vi "Autonomous Independent.vi"() -> ()   [LabVIEW 2012]
doc: "This VI is called when autonomous begins, and will automatically be terminated when autonomous ends. You can carry out timed or sensor driven robot movement independently without needing to return to the caller."
uses:
  <vilib>/Rock Robotics/WPI/Relay/WPI_RelayValue.ctl
  <vilib>/Rock Robotics/WPI/Solenoid/WPI_SolenoidValue.ctl
  Robot Global Data.vi
  <vilib>/Rock Robotics/WPI/RobotDrive/WPI_RobotDriveGetSetRefNum.vi
  <vilib>/Rock Robotics/WPI/Solenoid/WPI_SolenoidSetEnum.vi
  <vilib>/Rock Robotics/WPI/Joystick/WPI_JoystickGetSetRefNum.vi
panel:
  in  "Auton Launch Reduction":dbl
  in  "Quicklaunch State":T1(ring)
  in  "Fast-Slow Variable":dbl=1.0
  out "Launch Wait tick":dbl
  out "Time Between tick":dbl
  out "Charge Up tick":dbl
  in  "Time Between Launches":dbl=2000.0
  in  "Charge Up Time":dbl=4000.0
  in  "Launch Wait Time":dbl=500.0
  in  "Drive wait time corner":dbl
  in  "Drive wait time middle":dbl
  out "Field Position":enum16{"Corner", "Middle"}(ring)
  in  "Numeric 0":dbl
  out "Current Movement, for debugging":T2 {"Y Joystick Value" scale=1.0..-1.0; "X Joystick Value" scale=-1.0..1.0}
  in  "Array of robot movements":T3(array[cluster]) {"Y Joystick Value" scale=1.0..-1.0; "X Joystick Value" scale=-1.0..1.0}
  # "Be sure to right-click and choose Data Operations>>Make Current Value default if you want to save the array values with the VI"
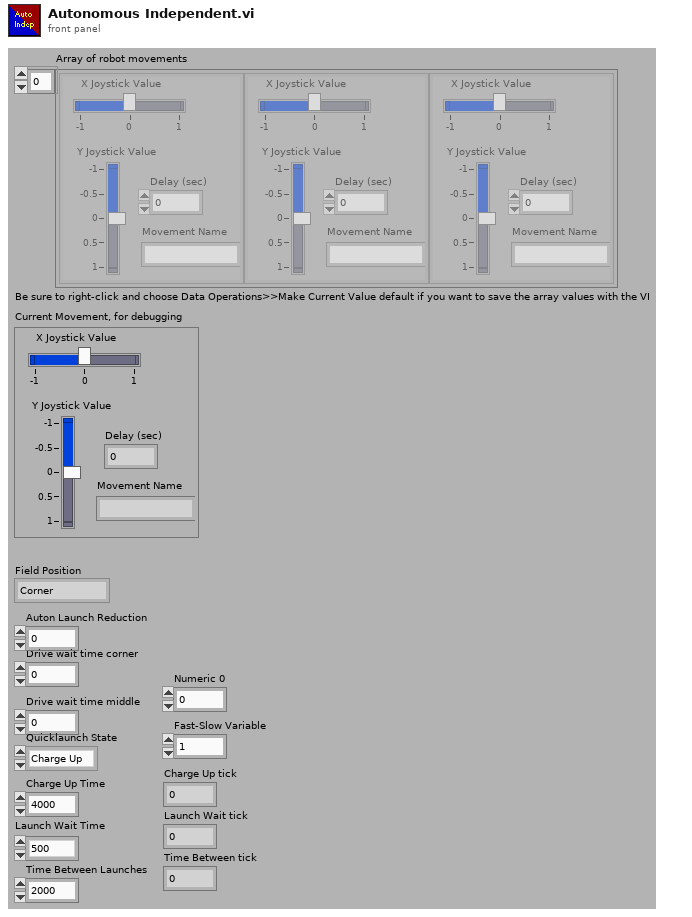
[diagram p1: front panel]
types:
  T1 = enum16{"Charge Up ", "Fire 1", "wait1", "Fire 2", "wait2", "Fire 3", "wait3", "Fire 4"}
  T2 = cluster{"X Joystick Value":dbl, "Y Joystick Value":dbl, "Delay (sec)":dbl, "Movement Name":string}
  T3 = cluster{"X Joystick Value":dbl, "Y Joystick Value":dbl, "Delay (sec)":dbl, "Movement Name":string}[]
  T4 = typedef "WPI_JoystickDevRef.ctl" = cluster{"Device":T5}
  T5 = typedef "WPI_JoystickDeviceEnum.ctl" = enum16{"USB 1", "USB 2", "USB 3", "USB 4", "Kinect 1", "Kinect 2"}
  T6 = cluster{"axis 1 (x)":dbl, "axis 2 (y)":dbl, "axis 3 (throttle)":dbl, "axis 4":dbl, "axis 5":dbl, "axis 6":dbl}
  T7 = typedef "WPI_SolenoidValue.ctl" = enum16{"Off", "On", "Forward", "Reverse"}
  T8 = typedef "WPI_RobotDriveDevRef.ctl" = cluster{"DevStatus":errorcluster, "Motors[]":T9[], "Square Inputs":bool, "Max Output":dbl, "Isochronous":bool}
  T9 = typedef "WPI_MotorControlDeviceRef.ctl" = cluster{"DeviceStatus":errorcluster, "Type":enum16{"PWM", "CAN"}, "PWM":cluster{"Digital Module":T10, "PWM Channel":T11, "DeadBand":T12}, "CAN":cluster{"Device Number":u8, "Control Mode":T13, "Semaphore":T14, "Max Vout":dbl}, "Invert":bool, "TransformRef":T15, "InvTransformRef":T15}
  T10 = typedef "FPGA_TypedefDigitalModule.ctl" = enum16{"Digital Module 1", "Digital Module 2"}
  T11 = typedef "FPGA_DIOPWMChannel.ctl" = enum8{"PWM 1", "PWM 2", "PWM 3", "PWM 4", "PWM 5", "PWM 6", "PWM 7", "PWM 8", "PWM 9", "PWM 10", "Invalid"}
  T12 = typedef "WPI_PWMDeadband.ctl" = cluster{"Name":string, "maxPositivePwm":i32, "minPositivePwm":i32, "centerPwm":i32, "maxNegativePwm":i32, "minNegativePwm":i32, "angularRange":u16}
  T13 = typedef "WPI_CANJaguar_ControlMode.ctl" = enum8{"Percent VBus", "Current", "Speed", "Position", "Voltage"}
  T14 = typedef "Semaphore RefNum" = refnum<k1>
  T15 = typedef "WPI_PWMTransform_ConPane.ctl" = refnum<vi>
  T16 = typedef "WPI_SolenoidDevRef.ctl" = cluster{"DevStatus":errorcluster, "Solenoid Module":T17, "Forward Solenoid Channel":T18, "Reverse Solenoid Channel":T18}
  T17 = typedef "FPGA_TypedefSolenoidModule.ctl" = enum16{"Solenoid Module 1", "Solenoid Module 2"}
  T18 = typedef "WPI_SolenoidChannel.ctl" = enum8{"Solenoid 1", "Solenoid 2", "Solenoid 3", "Solenoid 4", "Solenoid 5", "Solenoid 6", "Solenoid 7", "Solenoid 8", "Invalid"}
  T19 = typedef "WPI_RelayValue.ctl" = enum16{"Off", "On", "Forward", "Reverse"}
  T20 = typedef "WPI_RelayDevRef.ctl" = cluster{"DevStatus":errorcluster, "Relay Channel":T21, "Digital Module":T10, "Relay Direction":T22}
  T21 = typedef "FPGA_DIORelayChannel.ctl" = enum8{"Relay 1", "Relay 2", "Relay 3", "Relay 4", "Relay 5", "Relay 6", "Relay 7", "Relay 8", "Invalid"}
  T22 = typedef "WPI_RelayDirection.ctl" = enum16{"Both directions", "Forward only", "Reverse only"}
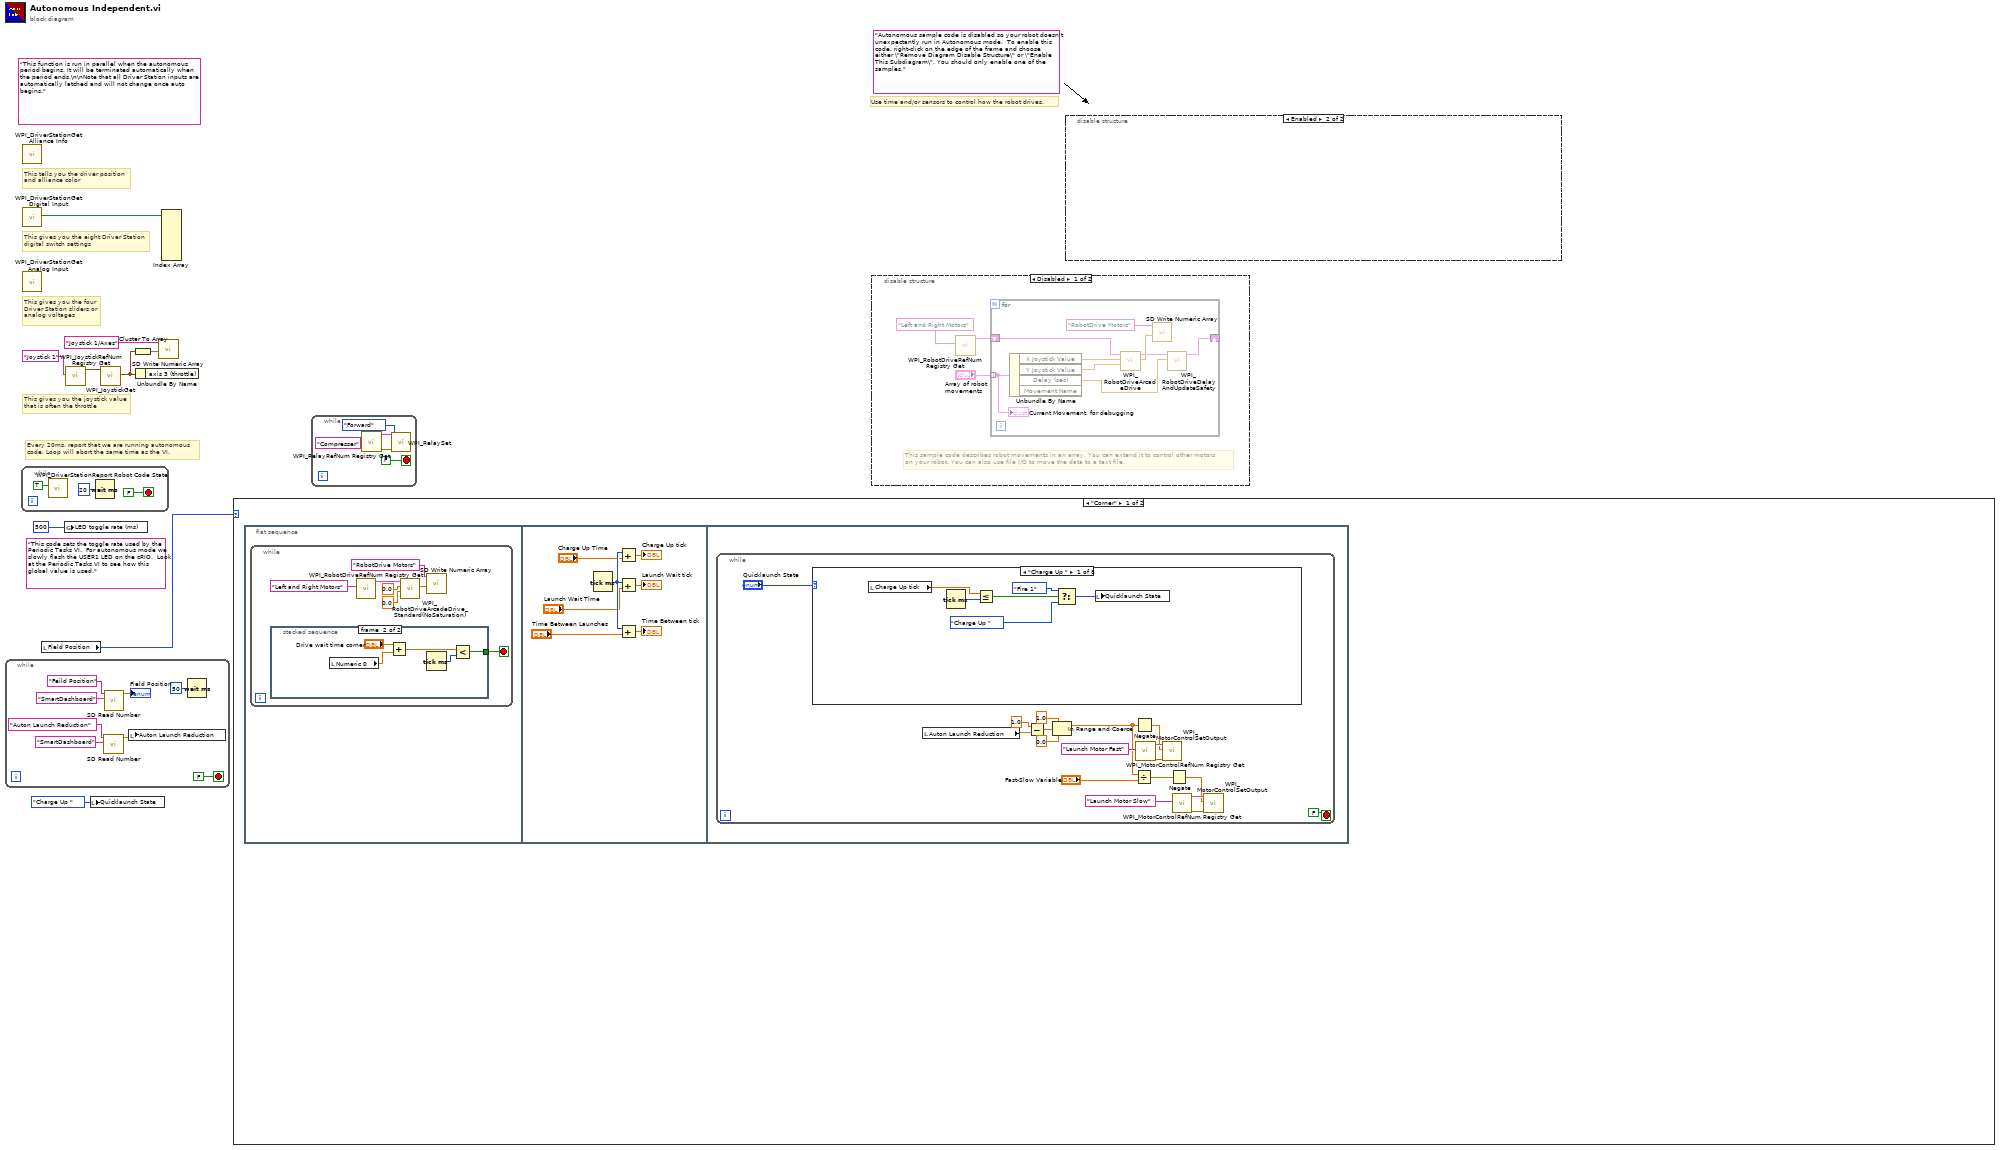
[diagram p0: block diagram]
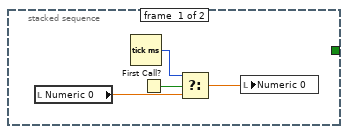
[diagram p2: hidden frame]
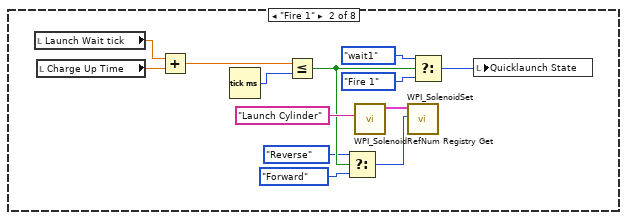
[diagram p3: hidden frame]
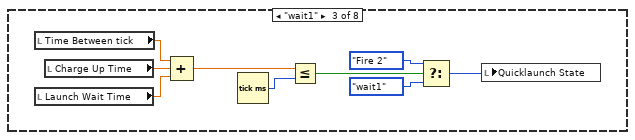
[diagram p4: hidden frame]
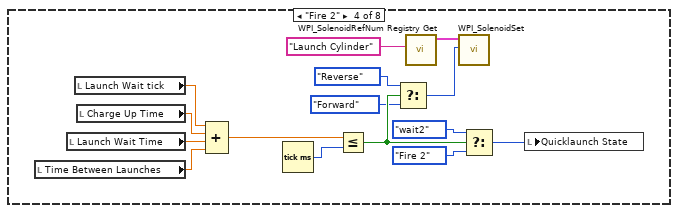
[diagram p5: hidden frame]
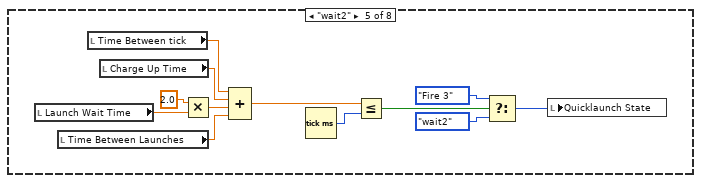
[diagram p6: hidden frame]
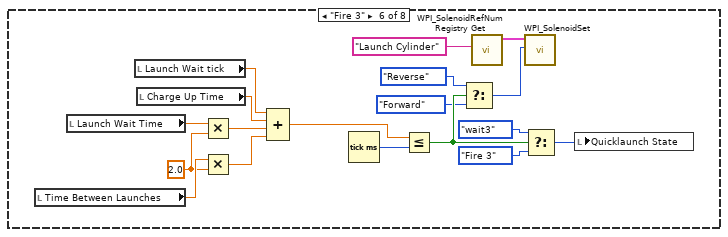
[diagram p7: hidden frame]
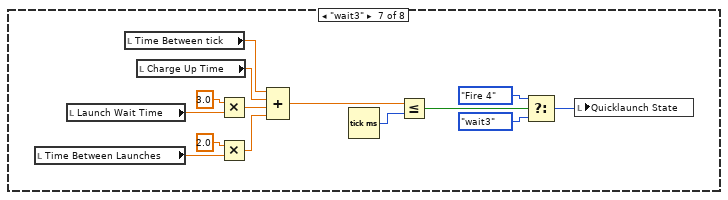
[diagram p8: hidden frame]
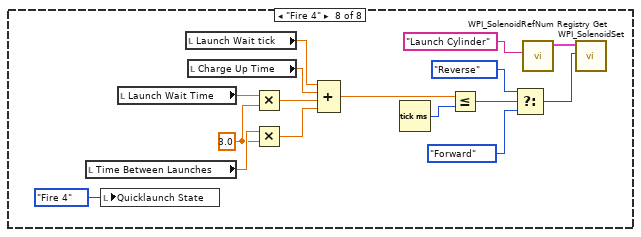
[diagram p9: hidden frame]
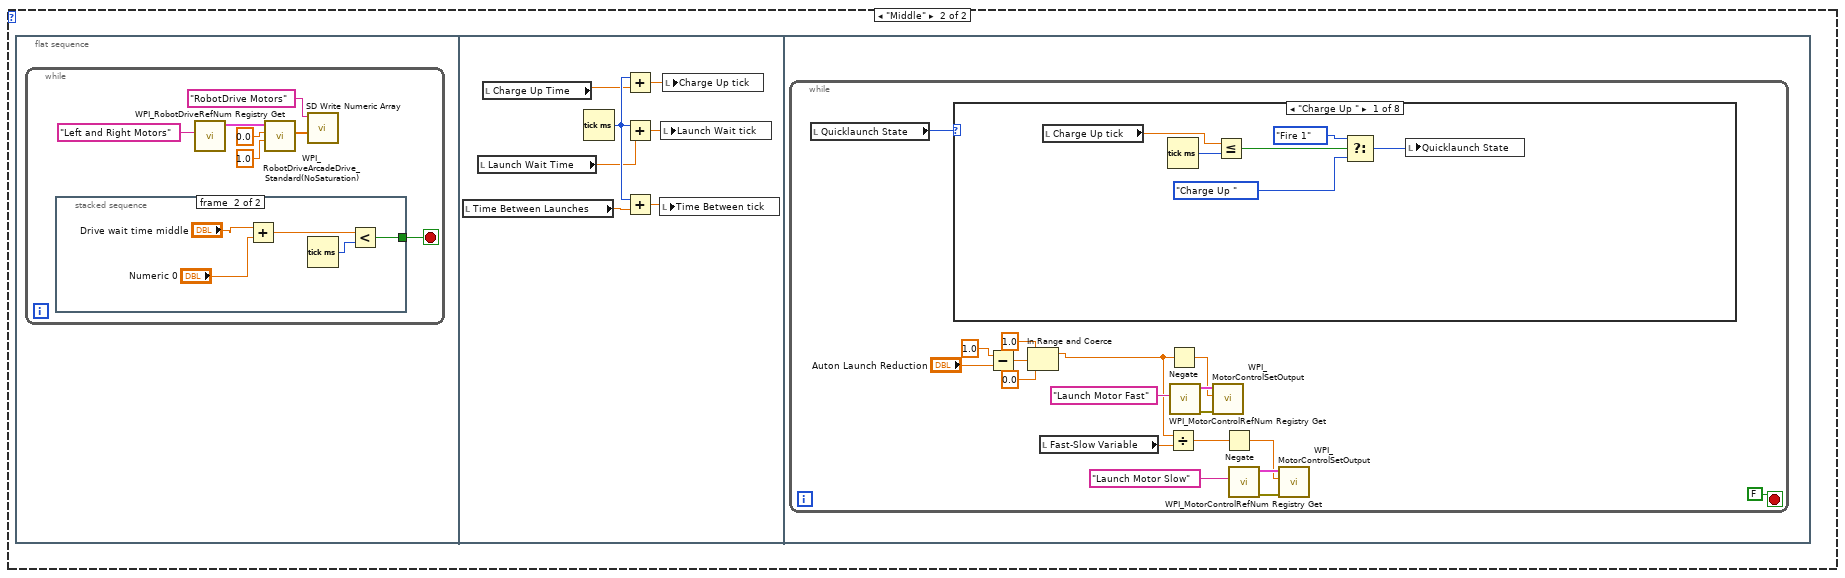
[diagram p10: hidden frame]
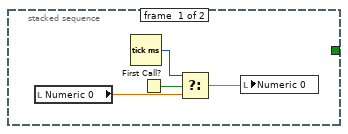
[diagram p11: hidden frame]
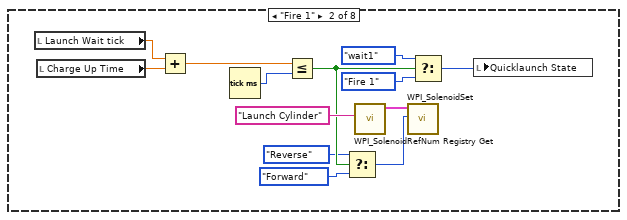
[diagram p12: hidden frame]
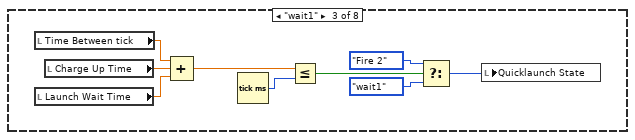
[diagram p13: hidden frame]
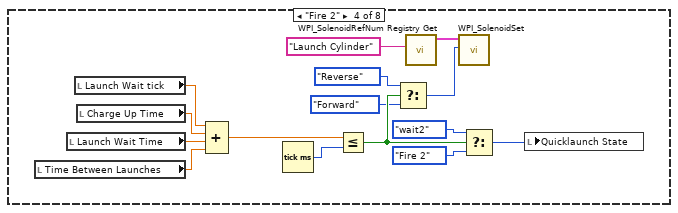
[diagram p14: hidden frame]
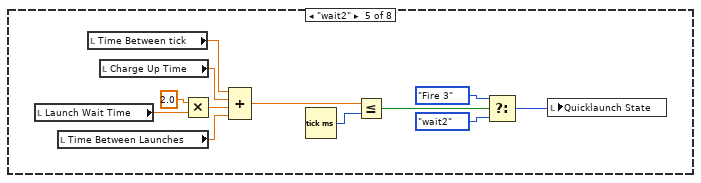
[diagram p15: hidden frame]
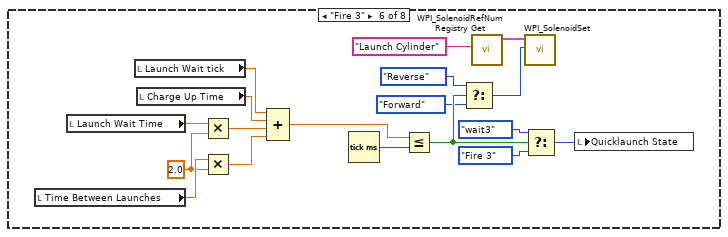
[diagram p16: hidden frame]
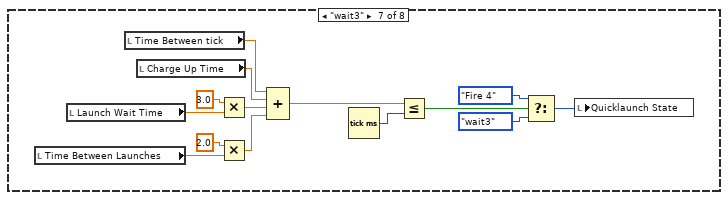
[diagram p17: hidden frame]
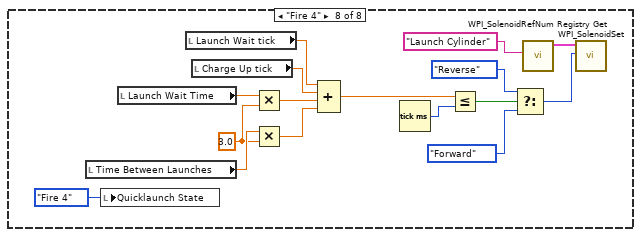
[diagram p18: hidden frame]
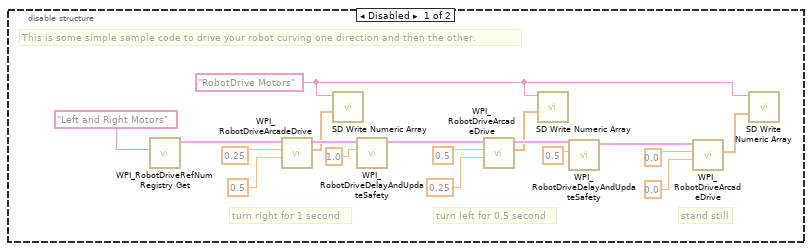
[diagram p20: hidden frame]
diagram:
  (unwired) "This code sets the toggle rate used by the Periodic Tasks VI.  For autonomous mode we slowly flash the USER1 LED on the cRIO.  Look at the Periodic Tasks VI to see how this global value is used."
  (unwired) "Autonomous sample code is disabled so your robot doesn't unexpectantly run in Autonomous mode.  To enable this code, right-click on the edge of the frame and choose either \"Remove Diagram Disable Structure\" or \"Enable This Subdiagram\". You should only enable one of the samples."
  (unwired) "This function is run in parallel when the autonomous period begins. It will be terminated automatically when the period ends.\n\nNote that all Driver Station inputs are automatically latched and will not change once auto begins."
  # "Every 20ms, report that we are running autonomous\ncode. Loop will abort the same time as the VI."
  # "This gives you the joystick value\nthat is often the throttle"
  # "Use time and/or sensors to control how the robot drives."
  # "This tells you the driver position\nand alliance color"
  # "This gives you the eight Driver Station\ndigital switch settings"
  # "This gives you the four\nDriver Station sliders or\nanalog voltages"
  n1 = while {
    stop <- FALSE stop-if-true
    n2 = call <vilib>:"SD Read Number.vi"("Table Prefix"="SmartDashboard", "Name"="Auton Launch Reduction") -> ("Numeric"=w12:dbl)  [unwired: 7 in, 2 out]
    n3 = call <vilib>:"SD Read Number.vi"("Table Prefix"="SmartDashboard", "Name"="Feild Position") -> ("Numeric"=→"Field Position":dbl)  [unwired: 7 in, 2 out]
    n4 = local write "Auton Launch Reduction"(w12) -> ()
    n5 = Wait (ms)(milliseconds to wait=u32 50) -> ()  [unwired: 1 out]
  }
  n6 = while {
    stop <- FALSE stop-if-true
    n7 = call <vilib>:"WPI_DriverStationReport Robot Code State.vi"("Autonomous"=TRUE) -> ()  [unwired: 10 in, 1 out]
    n8 = Wait (ms)(milliseconds to wait=u32 20) -> ()  [unwired: 1 out]
  }
  n9 = call <vilib>:"WPI_DriverStationGet Alliance Info.vi"() -> ()  [unwired: 12 out]
  n10 = call <vilib>:"WPI_DriverStationGet Digital Input.vi"() -> ("Driver Station Digital Input (1-8)"=w9:bool[])  [unwired: 11 out]
  n11 = call <vilib>:"WPI_DriverStationGet Analog Input.vi"() -> ()  [unwired: 12 out]
  n12 = local read "Field Position"() -> (w2:enum16{"Corner", "Middle"})
  n13 = global write "Robot Global Data.vi" "LED toggle rate (ms)"(u32 500 ("LED ms toggle rate")) -> ()
  n14 = call <vilib>:"WPI_JoystickRefNum Registry Get.vi"("refnum name"="Joystick 1") -> ("JoystickDevRef"=w7:T4)  [unwired: 1 in, 9 out]
  n15 = local write "Quicklaunch State"(T1."Charge Up " ("Quicklaunch State")) -> ()
  n16 = call <vilib>:"WPI_JoystickGet.vi"("JoystickDevRef"=w7) -> ("Axes"=w4:T6)  [unwired: 1 in, 5 out]
  n17 = Cluster To Array(cluster=w4) -> (array=w5:dbl[])
  n18 = Unbundle By Name(w4) -> ()  [unwired: 1 out]
  n19 = call <vilib>:"SD Write Numeric Array.vi"("Numeric Array"=w5, "Name"="Joystick 1/Axes") -> ()  [unwired: 8 in, 2 out]
  n20 = Index Array(array=w9) -> ()  [unwired: 8 in, 8 out]
  n21 = case shown="\"Corner\"" w2 {
    frame "Corner" {
      n22 = flat-sequence {
        frame #0 {
          n23 = while {
            stop <- w21 stop-if-true
            n24 = stacked-sequence {
              tunnel: [_ w33] -> w21
              frame #0 {
                n25 = local read "Numeric 0"() -> (w29:dbl)
                n26 = Tick Count (ms)() -> (millisecond timer value=w30:u32)
                n27 = First Call?() -> (First Call?: T/F=w31:bool)
                n28 = Select(t=w30, s=w31, f=w29) -> (s? t:f=w28:dbl)
                n29 = local write "Numeric 0"(w28) -> ()
              }
              frame #1 {
                n30 = local read "Numeric 0"() -> (w36:dbl)
                n31 = Add(x="Drive wait time corner", y=w36) -> (x+y=w35:dbl)
                n32 = Tick Count (ms)() -> (millisecond timer value=w34:u32)
                n33 = Less?(x=w35, y=w34) -> (x < y?=w33:bool)
              }
            }
            n34 = call <vilib>:"WPI_RobotDriveRefNum Registry Get.vi"("refnum name"="Left and Right Motors") -> ("RobotDriveDevRef"=w26:T8)  [unwired: 1 in, 9 out]
            n35 = call <vilib>:"WPI_RobotDriveArcadeDrive_Standard(NoSaturation).vi"("Y axis value"=0.0 ("X axis value"), "X axis value"=0.0, "RobotDriveDevRef"=w26) -> ("Motor Values"=w24:dbl[])  [unwired: 1 in, 7 out]
            n36 = call <vilib>:"SD Write Numeric Array.vi"("Numeric Array"=w24, "Name"="RobotDrive Motors") -> ()  [unwired: 8 in, 2 out]
          }
        }
        frame #1 {
          n37 = Tick Count (ms)() -> (millisecond timer value=w40:u32)
          n38 = Add(x=w40, y="Charge Up Time") -> (x+y=→"Charge Up tick":dbl)
          n39 = Add(x=w40, y="Launch Wait Time") -> (x+y=→"Launch Wait tick":dbl)
          n40 = Add(x=w40, y="Time Between Launches") -> (x+y=→"Time Between tick":dbl)
        }
        frame #2 {
          n41 = while {
            stop <- FALSE stop-if-true
            n42 = case shown="\"Charge Up \"" "Quicklaunch State" {
              frame "Charge Up " {
                n43 = local read "Charge Up tick"() -> (w62:dbl)
                n44 = Tick Count (ms)() -> (millisecond timer value=w66:u32)
                n45 = Less Or Equal?(x=w62, y=w66) -> (x <= y?=w65:bool)
                n46 = Select(t=T1."Fire 1", s=w65, f=T1."Charge Up ") -> (s? t:f=w67:T1)
                n47 = local write "Quicklaunch State"(w67) -> ()
              }
              frame "Fire 1" {
                n48 = local read "Launch Wait tick"() -> (w76:dbl)
                n49 = local read "Charge Up Time"() -> (w74:dbl)
                n50 = Add(x=w76, y=w74) -> (x+y=w75:dbl)
                n51 = Tick Count (ms)() -> (millisecond timer value=w80:u32)
                n52 = Less Or Equal?(x=w75, y=w80) -> (x <= y?=w71:bool)
                n53 = Select(t=WPI_SolenoidValue."Reverse" ("Value"), s=w71, f=WPI_SolenoidValue."Forward" ("Value")) -> (s? t:f=w68:T7)
                n54 = call <vilib>:"WPI_SolenoidRefNum Registry Get.vi"("refnum name"="Launch Cylinder") -> ("SolenoidDevRef"=w73:T16)  [unwired: 9 in, 1 out]
                n55 = call-poly <vilib>:"WPI_SolenoidSet.vi"("Value"=w68, "SolenoidDevRef"=w73) -> ()  [unwired: 8 in, 2 out]
                n56 = Select(t=T1."wait1", s=w71, f=T1."Fire 1") -> (s? t:f=w79:T1)
                n57 = local write "Quicklaunch State"(w79) -> ()
              }
              frame "wait1" {
                n58 = local read "Time Between tick"() -> (w82:dbl)
                n59 = local read "Launch Wait Time"() -> (w83:dbl)
                n60 = local read "Charge Up Time"() -> (w84:dbl)
                n61 = Compound Arithmetic op=ADD(w82, w84, w83) -> (w81:dbl)
                n62 = Tick Count (ms)() -> (millisecond timer value=w86:u32)
                n63 = Less Or Equal?(x=w81, y=w86) -> (x <= y?=w85:bool)
                n64 = Select(t=T1."Fire 2", s=w85, f=T1."wait1") -> (s? t:f=w89:T1)
                n65 = local write "Quicklaunch State"(w89) -> ()
              }
              frame "Fire 2" {
                n66 = local read "Time Between Launches"() -> (w91:dbl)
                n67 = local read "Launch Wait Time"() -> (w92:dbl)
                n68 = local read "Launch Wait tick"() -> (w94:dbl)
                n69 = local read "Charge Up Time"() -> (w93:dbl)
                n70 = Compound Arithmetic op=ADD(w94, w93, w92, w91) -> (w90:dbl)
                n71 = Tick Count (ms)() -> (millisecond timer value=w104:u32)
                n72 = Less Or Equal?(x=w90, y=w104) -> (x <= y?=w98:bool)
                n73 = Select(t=WPI_SolenoidValue."Reverse" ("Value"), s=w98, f=WPI_SolenoidValue."Forward" ("Value")) -> (s? t:f=w95:T7)
                n74 = call <vilib>:"WPI_SolenoidRefNum Registry Get.vi"("refnum name"="Launch Cylinder") -> ("SolenoidDevRef"=w100:T16)  [unwired: 9 in, 1 out]
                n75 = call-poly <vilib>:"WPI_SolenoidSet.vi"("Value"=w95, "SolenoidDevRef"=w100) -> ()  [unwired: 8 in, 2 out]
                n76 = Select(t=T1."wait2", s=w98, f=T1."Fire 2") -> (s? t:f=w103:T1)
                n77 = local write "Quicklaunch State"(w103) -> ()
              }
              frame "wait2" {
                n78 = local read "Launch Wait Time"() -> (w110:dbl)
                n79 = local read "Time Between Launches"() -> (w107:dbl)
                n80 = local read "Time Between tick"() -> (w109:dbl)
                n81 = local read "Charge Up Time"() -> (w111:dbl)
                n82 = Multiply(x=2.0, y=w110) -> (x*y=w106:dbl)
                n83 = Compound Arithmetic op=ADD(w109, w111, w106, w107) -> (w108:dbl)
                n84 = Tick Count (ms)() -> (millisecond timer value=w113:u32)
                n85 = Less Or Equal?(x=w108, y=w113) -> (x <= y?=w112:bool)
                n86 = Select(t=T1."Fire 3", s=w112, f=T1."wait2") -> (s? t:f=w116:T1)
                n87 = local write "Quicklaunch State"(w116) -> ()
              }
              frame "Fire 3" {
                w117 = 2.0 ("y")
                n88 = local read "Time Between Launches"() -> (w120:dbl)
                n89 = local read "Launch Wait Time"() -> (w121:dbl)
                n90 = local read "Launch Wait tick"() -> (w124:dbl)
                n91 = local read "Charge Up Time"() -> (w123:dbl)
                n92 = Multiply(x=w121, y=w117) -> (x*y=w118:dbl)
                n93 = Multiply(x=w120, y=w117) -> (x*y=w119:dbl)
                n94 = Compound Arithmetic op=ADD(w124, w123, w118, w119) -> (w122:dbl)
                n95 = Tick Count (ms)() -> (millisecond timer value=w134:u32)
                n96 = Less Or Equal?(x=w122, y=w134) -> (x <= y?=w128:bool)
                n97 = Select(t=WPI_SolenoidValue."Reverse" ("Value"), s=w128, f=WPI_SolenoidValue."Forward" ("Value")) -> (s? t:f=w125:T7)
                n98 = call <vilib>:"WPI_SolenoidRefNum Registry Get.vi"("refnum name"="Launch Cylinder") -> ("SolenoidDevRef"=w130:T16)  [unwired: 9 in, 1 out]
                n99 = call-poly <vilib>:"WPI_SolenoidSet.vi"("Value"=w125, "SolenoidDevRef"=w130) -> ()  [unwired: 8 in, 2 out]
                n100 = Select(t=T1."wait3", s=w128, f=T1."Fire 3") -> (s? t:f=w133:T1)
                n101 = local write "Quicklaunch State"(w133) -> ()
              }
              frame "wait3" {
                n102 = local read "Time Between Launches"() -> (w139:dbl)
                n103 = local read "Launch Wait Time"() -> (w142:dbl)
                n104 = local read "Time Between tick"() -> (w141:dbl)
                n105 = local read "Charge Up Time"() -> (w143:dbl)
                n106 = Multiply(x=3.0, y=w142) -> (x*y=w138:dbl)
                n107 = Multiply(x=2.0, y=w139) -> (x*y=w136:dbl)
                n108 = Compound Arithmetic op=ADD(w141, w143, w138, w136) -> (w140:dbl)
                n109 = Tick Count (ms)() -> (millisecond timer value=w145:u32)
                n110 = Less Or Equal?(x=w140, y=w145) -> (x <= y?=w144:bool)
                n111 = Select(t=T1."Fire 4", s=w144, f=T1."wait3") -> (s? t:f=w148:T1)
                n112 = local write "Quicklaunch State"(w148) -> ()
              }
              frame "Fire 4" {
                w150 = 3.0 ("y")
                n113 = local read "Time Between Launches"() -> (w153:dbl)
                n114 = local write "Quicklaunch State"(T1."Fire 4" ("Quicklaunch State")) -> ()
                n115 = local read "Launch Wait Time"() -> (w154:dbl)
                n116 = local read "Launch Wait tick"() -> (w157:dbl)
                n117 = local read "Charge Up Time"() -> (w156:dbl)
                n118 = Multiply(x=w154, y=w150) -> (x*y=w151:dbl)
                n119 = Multiply(x=w153, y=w150) -> (x*y=w152:dbl)
                n120 = Compound Arithmetic op=ADD(w157, w156, w151, w152) -> (w155:dbl)
                n121 = Tick Count (ms)() -> (millisecond timer value=w164:u32)
                n122 = Less Or Equal?(x=w155, y=w164) -> (x <= y?=w161:bool)
                n123 = Select(t=WPI_SolenoidValue."Reverse" ("Value"), s=w161, f=WPI_SolenoidValue."Forward" ("Value")) -> (s? t:f=w158:T7)
                n124 = call <vilib>:"WPI_SolenoidRefNum Registry Get.vi"("refnum name"="Launch Cylinder") -> ("SolenoidDevRef"=w163:T16)  [unwired: 9 in, 1 out]
                n125 = call-poly <vilib>:"WPI_SolenoidSet.vi"("Value"=w158, "SolenoidDevRef"=w163) -> ()  [unwired: 8 in, 2 out]
              }
            }
            n126 = local read "Auton Launch Reduction"() -> (w44:dbl)
            n127 = Subtract(x=1.0, y=w44) -> (x-y=w48:dbl)
            n128 = In Range and Coerce(upper limit=1.0, x=w48, lower limit=0.0 ("x")) -> (coerced(x)=w45:dbl)  [unwired: 1 out]
            n129 = Divide(x=w45, y="Fast-Slow Variable") -> (x/y=w53:dbl)
            n130 = Negate(x=w45) -> (-x=w52:dbl)
            n131 = call <vilib>:"WPI_MotorControlRefNum Registry Get.vi"("refnum name"="Launch Motor Fast") -> ("error out"=w55:errorcluster, "MotorControlDevRef"=w56:T9)  [unwired: 9 in]
            n132 = call <vilib>:"WPI_MotorControlSetOutput.vi"("error in (no error)"=w55, "Output"=w52, "MotorControlDevRef"=w56) -> ()  [unwired: 6 in, 3 out]
            n133 = Negate(x=w53) -> (-x=w51:dbl)
            n134 = call <vilib>:"WPI_MotorControlRefNum Registry Get.vi"("refnum name"="Launch Motor Slow") -> ("error out"=w58:errorcluster, "MotorControlDevRef"=w57:T9)  [unwired: 9 in]
            n135 = call <vilib>:"WPI_MotorControlSetOutput.vi"("error in (no error)"=w58, "Output"=w51, "MotorControlDevRef"=w57) -> ()  [unwired: 6 in, 3 out]
          }
        }
      }
    }
    frame "Middle" {
      n136 = flat-sequence {
        frame #0 {
          n137 = while {
            stop <- w165 stop-if-true
            n138 = stacked-sequence {
              tunnel: [_ w178] -> w165
              frame #0 {
                n139 = local read "Numeric 0"() -> (w173:dbl)
                n140 = Tick Count (ms)() -> (millisecond timer value=w174:u32)
                n141 = First Call?() -> (First Call?: T/F=w175:bool)
                n142 = Select(t=w174, s=w175, f=w173) -> (s? t:f=w172:dbl)
                n143 = local write "Numeric 0"(w172) -> ()
              }
              frame #1 {
                n144 = Add(x="Drive wait time middle", y="Numeric 0") -> (x+y=w180:dbl)
                n145 = Tick Count (ms)() -> (millisecond timer value=w179:u32)
                n146 = Less?(x=w180, y=w179) -> (x < y?=w178:bool)
              }
            }
            n147 = call <vilib>:"WPI_RobotDriveRefNum Registry Get.vi"("refnum name"="Left and Right Motors") -> ("RobotDriveDevRef"=w170:T8)  [unwired: 1 in, 9 out]
            n148 = call <vilib>:"WPI_RobotDriveArcadeDrive_Standard(NoSaturation).vi"("Y axis value"=1.0 ("X axis value"), "X axis value"=0.0, "RobotDriveDevRef"=w170) -> ("Motor Values"=w168:dbl[])  [unwired: 1 in, 7 out]
            n149 = call <vilib>:"SD Write Numeric Array.vi"("Numeric Array"=w168, "Name"="RobotDrive Motors") -> ()  [unwired: 8 in, 2 out]
          }
        }
        frame #1 {
          n150 = local read "Time Between Launches"() -> (w184:dbl)
          n151 = local read "Launch Wait Time"() -> (w185:dbl)
          n152 = local read "Charge Up Time"() -> (w186:dbl)
          n153 = Tick Count (ms)() -> (millisecond timer value=w187:u32)
          n154 = Add(x=w187, y=w186) -> (x+y=w181:dbl)
          n155 = Add(x=w187, y=w185) -> (x+y=w182:dbl)
          n156 = Add(x=w187, y=w184) -> (x+y=w183:dbl)
          n157 = local write "Time Between tick"(w183) -> ()
          n158 = local write "Launch Wait tick"(w182) -> ()
          n159 = local write "Charge Up tick"(w181) -> ()
        }
        frame #2 {
          n160 = while {
            stop <- FALSE stop-if-true
            n161 = local read "Quicklaunch State"() -> (w195:T1)
            n162 = case shown="\"Charge Up \"" w195 {
              frame "Charge Up " {
                n163 = local read "Charge Up tick"() -> (w206:dbl)
                n164 = Tick Count (ms)() -> (millisecond timer value=w210:u32)
                n165 = Less Or Equal?(x=w206, y=w210) -> (x <= y?=w209:bool)
                n166 = Select(t=T1."Fire 1", s=w209, f=T1."Charge Up ") -> (s? t:f=w211:T1)
                n167 = local write "Quicklaunch State"(w211) -> ()
              }
              frame "Fire 1" {
                n168 = local read "Launch Wait tick"() -> (w220:dbl)
                n169 = local read "Charge Up Time"() -> (w218:dbl)
                n170 = Add(x=w220, y=w218) -> (x+y=w219:dbl)
                n171 = Tick Count (ms)() -> (millisecond timer value=w224:u32)
                n172 = Less Or Equal?(x=w219, y=w224) -> (x <= y?=w215:bool)
                n173 = Select(t=WPI_SolenoidValue."Reverse" ("Value"), s=w215, f=WPI_SolenoidValue."Forward" ("Value")) -> (s? t:f=w212:T7)
                n174 = call <vilib>:"WPI_SolenoidRefNum Registry Get.vi"("refnum name"="Launch Cylinder") -> ("SolenoidDevRef"=w217:T16)  [unwired: 9 in, 1 out]
                n175 = call-poly <vilib>:"WPI_SolenoidSet.vi"("Value"=w212, "SolenoidDevRef"=w217) -> ()  [unwired: 8 in, 2 out]
                n176 = Select(t=T1."wait1", s=w215, f=T1."Fire 1") -> (s? t:f=w223:T1)
                n177 = local write "Quicklaunch State"(w223) -> ()
              }
              frame "wait1" {
                n178 = local read "Time Between tick"() -> (w227:dbl)
                n179 = local read "Launch Wait Time"() -> (w225:dbl)
                n180 = local read "Charge Up Time"() -> (w228:dbl)
                n181 = Compound Arithmetic op=ADD(w227, w228, w225) -> (w226:dbl)
                n182 = Tick Count (ms)() -> (millisecond timer value=w230:u32)
                n183 = Less Or Equal?(x=w226, y=w230) -> (x <= y?=w229:bool)
                n184 = Select(t=T1."Fire 2", s=w229, f=T1."wait1") -> (s? t:f=w233:T1)
                n185 = local write "Quicklaunch State"(w233) -> ()
              }
              frame "Fire 2" {
                n186 = local read "Time Between Launches"() -> (w235:dbl)
                n187 = local read "Launch Wait Time"() -> (w236:dbl)
                n188 = local read "Launch Wait tick"() -> (w238:dbl)
                n189 = local read "Charge Up Time"() -> (w237:dbl)
                n190 = Compound Arithmetic op=ADD(w238, w237, w236, w235) -> (w234:dbl)
                n191 = Tick Count (ms)() -> (millisecond timer value=w248:u32)
                n192 = Less Or Equal?(x=w234, y=w248) -> (x <= y?=w242:bool)
                n193 = Select(t=WPI_SolenoidValue."Reverse" ("Value"), s=w242, f=WPI_SolenoidValue."Forward" ("Value")) -> (s? t:f=w239:T7)
                n194 = call <vilib>:"WPI_SolenoidRefNum Registry Get.vi"("refnum name"="Launch Cylinder") -> ("SolenoidDevRef"=w244:T16)  [unwired: 9 in, 1 out]
                n195 = call-poly <vilib>:"WPI_SolenoidSet.vi"("Value"=w239, "SolenoidDevRef"=w244) -> ()  [unwired: 8 in, 2 out]
                n196 = Select(t=T1."wait2", s=w242, f=T1."Fire 2") -> (s? t:f=w247:T1)
                n197 = local write "Quicklaunch State"(w247) -> ()
              }
              frame "wait2" {
                n198 = local read "Launch Wait Time"() -> (w254:dbl)
                n199 = local read "Time Between Launches"() -> (w251:dbl)
                n200 = local read "Time Between tick"() -> (w253:dbl)
                n201 = local read "Charge Up Time"() -> (w255:dbl)
                n202 = Multiply(x=2.0, y=w254) -> (x*y=w250:dbl)
                n203 = Compound Arithmetic op=ADD(w253, w255, w250, w251) -> (w252:dbl)
                n204 = Tick Count (ms)() -> (millisecond timer value=w257:u32)
                n205 = Less Or Equal?(x=w252, y=w257) -> (x <= y?=w256:bool)
                n206 = Select(t=T1."Fire 3", s=w256, f=T1."wait2") -> (s? t:f=w260:T1)
                n207 = local write "Quicklaunch State"(w260) -> ()
              }
              frame "Fire 3" {
                w261 = 2.0 ("y")
                n208 = local read "Time Between Launches"() -> (w264:dbl)
                n209 = local read "Launch Wait Time"() -> (w265:dbl)
                n210 = local read "Launch Wait tick"() -> (w268:dbl)
                n211 = local read "Charge Up Time"() -> (w267:dbl)
                n212 = Multiply(x=w265, y=w261) -> (x*y=w262:dbl)
                n213 = Multiply(x=w264, y=w261) -> (x*y=w263:dbl)
                n214 = Compound Arithmetic op=ADD(w268, w267, w262, w263) -> (w266:dbl)
                n215 = Tick Count (ms)() -> (millisecond timer value=w278:u32)
                n216 = Less Or Equal?(x=w266, y=w278) -> (x <= y?=w272:bool)
                n217 = Select(t=WPI_SolenoidValue."Reverse" ("Value"), s=w272, f=WPI_SolenoidValue."Forward" ("Value")) -> (s? t:f=w269:T7)
                n218 = call <vilib>:"WPI_SolenoidRefNum Registry Get.vi"("refnum name"="Launch Cylinder") -> ("SolenoidDevRef"=w274:T16)  [unwired: 9 in, 1 out]
                n219 = call-poly <vilib>:"WPI_SolenoidSet.vi"("Value"=w269, "SolenoidDevRef"=w274) -> ()  [unwired: 8 in, 2 out]
                n220 = Select(t=T1."wait3", s=w272, f=T1."Fire 3") -> (s? t:f=w277:T1)
                n221 = local write "Quicklaunch State"(w277) -> ()
              }
              frame "wait3" {
                n222 = local read "Time Between Launches"() -> (w283:dbl)
                n223 = local read "Launch Wait Time"() -> (w286:dbl)
                n224 = local read "Time Between tick"() -> (w285:dbl)
                n225 = local read "Charge Up Time"() -> (w287:dbl)
                n226 = Multiply(x=3.0, y=w286) -> (x*y=w282:dbl)
                n227 = Multiply(x=2.0, y=w283) -> (x*y=w280:dbl)
                n228 = Compound Arithmetic op=ADD(w285, w287, w282, w280) -> (w284:dbl)
                n229 = Tick Count (ms)() -> (millisecond timer value=w289:u32)
                n230 = Less Or Equal?(x=w284, y=w289) -> (x <= y?=w288:bool)
                n231 = Select(t=T1."Fire 4", s=w288, f=T1."wait3") -> (s? t:f=w292:T1)
                n232 = local write "Quicklaunch State"(w292) -> ()
              }
              frame "Fire 4" {
                w294 = 3.0 ("y")
                n233 = local read "Time Between Launches"() -> (w297:dbl)
                n234 = local write "Quicklaunch State"(T1."Fire 4" ("Quicklaunch State")) -> ()
                n235 = local read "Launch Wait Time"() -> (w298:dbl)
                n236 = local read "Launch Wait tick"() -> (w301:dbl)
                n237 = local read "Charge Up tick"() -> (w300:dbl)
                n238 = Multiply(x=w298, y=w294) -> (x*y=w295:dbl)
                n239 = Multiply(x=w297, y=w294) -> (x*y=w296:dbl)
                n240 = Compound Arithmetic op=ADD(w301, w300, w295, w296) -> (w299:dbl)
                n241 = Tick Count (ms)() -> (millisecond timer value=w308:u32)
                n242 = Less Or Equal?(x=w299, y=w308) -> (x <= y?=w305:bool)
                n243 = Select(t=WPI_SolenoidValue."Reverse" ("Value"), s=w305, f=WPI_SolenoidValue."Forward" ("Value")) -> (s? t:f=w302:T7)
                n244 = call <vilib>:"WPI_SolenoidRefNum Registry Get.vi"("refnum name"="Launch Cylinder") -> ("SolenoidDevRef"=w307:T16)  [unwired: 9 in, 1 out]
                n245 = call-poly <vilib>:"WPI_SolenoidSet.vi"("Value"=w302, "SolenoidDevRef"=w307) -> ()  [unwired: 8 in, 2 out]
              }
            }
            n246 = Subtract(x=1.0, y="Auton Launch Reduction") -> (x-y=w192:dbl)
            n247 = In Range and Coerce(upper limit=1.0, x=w192, lower limit=0.0 ("x")) -> (coerced(x)=w188:dbl)  [unwired: 1 out]
            n248 = local read "Fast-Slow Variable"() -> (w194:dbl)
            n249 = Divide(x=w188, y=w194) -> (x/y=w199:dbl)
            n250 = Negate(x=w188) -> (-x=w198:dbl)
            n251 = call <vilib>:"WPI_MotorControlRefNum Registry Get.vi"("refnum name"="Launch Motor Fast") -> ("error out"=w201:errorcluster, "MotorControlDevRef"=w202:T9)  [unwired: 9 in]
            n252 = call <vilib>:"WPI_MotorControlSetOutput.vi"("error in (no error)"=w201, "Output"=w198, "MotorControlDevRef"=w202) -> ()  [unwired: 6 in, 3 out]
            n253 = Negate(x=w199) -> (-x=w197:dbl)
            n254 = call <vilib>:"WPI_MotorControlRefNum Registry Get.vi"("refnum name"="Launch Motor Slow") -> ("error out"=w204:errorcluster, "MotorControlDevRef"=w203:T9)  [unwired: 9 in]
            n255 = call <vilib>:"WPI_MotorControlSetOutput.vi"("error in (no error)"=w204, "Output"=w197, "MotorControlDevRef"=w203) -> ()  [unwired: 6 in, 3 out]
          }
        }
      }
    }
  }
  n256 = while {
    stop <- FALSE stop-if-true
    n257 = call <vilib>:"WPI_RelayRefNum Registry Get.vi"("refnum name"="Compresser") -> ("error out"=w313:errorcluster, "RelayDevRef"=w312:T20)  [unwired: 9 in]
    n258 = call <vilib>:"WPI_RelaySet.vi"("error in (no error)"=w313, "RelayValue"=WPI_RelayValue."Forward", "RelayDevRef"=w312) -> ()  [unwired: 7 in, 2 out]
  }
  n259 = disable-structure shown="Disabled" {
    frame Disabled {
      # "This sample code describes robot movements in an array. You can extend it to control other motors\non your robot. You can also use file I/O to move the data to a text file."
      n260 = call <vilib>:"WPI_RobotDriveRefNum Registry Get.vi"("refnum name"="Left and Right Motors") -> ("RobotDriveDevRef"=w315:T8)  [unwired: 1 in, 9 out]
      n261 = for {
        shift-right: [w321] -> _
        shift-left: w315 -> [w322]
        tunnel: "Array of robot movements" -> [w317] mode=indexing
        n262 = Unbundle By Name(w317) -> ("X Joystick Value"=w320:dbl, "Y Joystick Value"=w319:dbl, "Delay (sec)"=w318:dbl)  [unwired: 1 out]
        n263 = call-poly <vilib>:"WPI_RobotDriveArcadeDrive.vi"("Y axis value"=w319, "X axis value"=w320, "RobotDriveDevRef"=w322) -> ("Motor Values"=w324:dbl[], "RobotDriveDevRef"=w323:T8)  [unwired: 1 in, 6 out]
        n264 = call <vilib>:"SD Write Numeric Array.vi"("Numeric Array"=w324, "Name"="RobotDrive Motors") -> ()  [unwired: 8 in, 2 out]
        n265 = call <vilib>:"WPI_RobotDriveDelayAndUpdateSafety.vi"("Delay (s)"=w318, "RobotDriveDevRef"=w323) -> ("RobotDriveDevRef 2"=w321:T8)  [unwired: 8 in, 1 out]
        "Current Movement, for debugging" <- w317
      }
    }
    frame Enabled {
    }
  }
  n266 = disable-structure shown="Enabled" {
    frame Disabled {
      w326 = "RobotDrive Motors" ("Name")
      # "This is some simple sample code to drive your robot curving one direction and then the other."
      # "stand still"
      # "turn left for 0.5 second"
      # "turn right for 1 second"
      n267 = call <vilib>:"WPI_RobotDriveRefNum Registry Get.vi"("refnum name"="Left and Right Motors") -> ("RobotDriveDevRef"=w330:T8)  [unwired: 1 in, 9 out]
      n268 = call-poly <vilib>:"WPI_RobotDriveArcadeDrive.vi"("Y axis value"=0.5 ("X axis value"), "X axis value"=0.25, "RobotDriveDevRef"=w330) -> ("Motor Values"=w329:dbl[], "RobotDriveDevRef"=w337:T8)  [unwired: 1 in, 6 out]
      n269 = call <vilib>:"SD Write Numeric Array.vi"("Numeric Array"=w329, "Name"=w326) -> ()  [unwired: 8 in, 2 out]
      n270 = call <vilib>:"WPI_RobotDriveDelayAndUpdateSafety.vi"("Delay (s)"=1.0, "RobotDriveDevRef"=w337) -> ("RobotDriveDevRef 2"=w336:T8)  [unwired: 8 in, 1 out]
      n271 = call-poly <vilib>:"WPI_RobotDriveArcadeDrive.vi"("Y axis value"=0.25 ("X axis value"), "X axis value"=0.5, "RobotDriveDevRef"=w336) -> ("Motor Values"=w328:dbl[], "RobotDriveDevRef"=w335:T8)  [unwired: 1 in, 6 out]
      n272 = call <vilib>:"SD Write Numeric Array.vi"("Numeric Array"=w328, "Name"=w326) -> ()  [unwired: 8 in, 2 out]
      n273 = call <vilib>:"WPI_RobotDriveDelayAndUpdateSafety.vi"("Delay (s)"=0.5, "RobotDriveDevRef"=w335) -> ("RobotDriveDevRef 2"=w334:T8)  [unwired: 8 in, 1 out]
      n274 = call-poly <vilib>:"WPI_RobotDriveArcadeDrive.vi"("Y axis value"=0.0 ("X axis value"), "X axis value"=0.0, "RobotDriveDevRef"=w334) -> ("Motor Values"=w327:dbl[])  [unwired: 1 in, 7 out]
      n275 = call <vilib>:"SD Write Numeric Array.vi"("Numeric Array"=w327, "Name"=w326) -> ()  [unwired: 8 in, 2 out]
    }
    frame Enabled {
    }
  }
